vi "Destroy.vi"(8 "Error In":errorcluster, 11 "Writer":refnum<class "Writer.lvclass">) -> (0 "Error Out":errorcluster)   [LabVIEW 2019, in "LabPack.lvlib" / "Writer.lvclass"]
doc: "Destroys an object of the Writer class. This must be called when shutting down an application to avoid memory leaks. This may free resources."
uses:
  Writer.lvclass
  Writer.lvclass/Writer.ctl
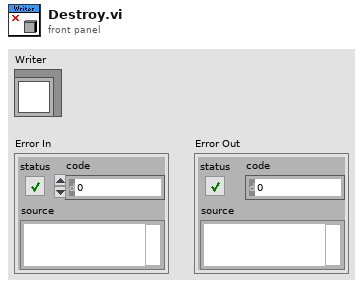
[diagram p1: front panel]
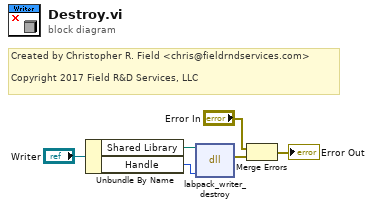
[diagram p0: block diagram]
diagram:
  # "Created by Christopher R. Field <chris@fieldrndservices.com>\n\nCopyright 2017 Field R&D Services, LLC"
  n1 = Unbundle By Name("Writer") -> ("Shared Library"=w5:path, "Handle"=w4:u64)
  n2 = dll-call lib="D:/Users/cfield/Code/MessagePack/LabPack/LabVIEW/trunk/src/LabPack/Private/labpack-x64.dll" fn="labpack_writer_destroy"(path in=w5, "writer"=w4) -> (error out=w1:errorcluster)  [unwired: 4 in, 1 out]
  n3 = Merge Errors("Error In", w1) -> (→"Error Out":errorcluster)
